vi "803M超标留样MB通讯.vi"(8 "error in (no error)":errorcluster, 9 "VISA resource name":refnum<visa-resource-name> caption="VISA资源名称", 10 "data_in":T1, 11 "功能输入":T2(ring)) -> (0 "error out":errorcluster, 2 "data_out":cluster{"Registers":u16[], "Coils":bool[]})   [LabVIEW 2016, in "超标留样集成.lvlib" / "德润DR803M超标留样.lvlib"]
uses:
  <vilib>/Plasmionique/MB Master/MB_Master_Serial/MB_Master_Serial.lvclass
  D:/Program Files (x86)/National Instruments/LabVIEW 2016/vi.lib/Plasmionique/MB Master/MB_Master/MB_Master.lvclass
  <vilib>/Plasmionique/MB Master/MB Master.lvlib
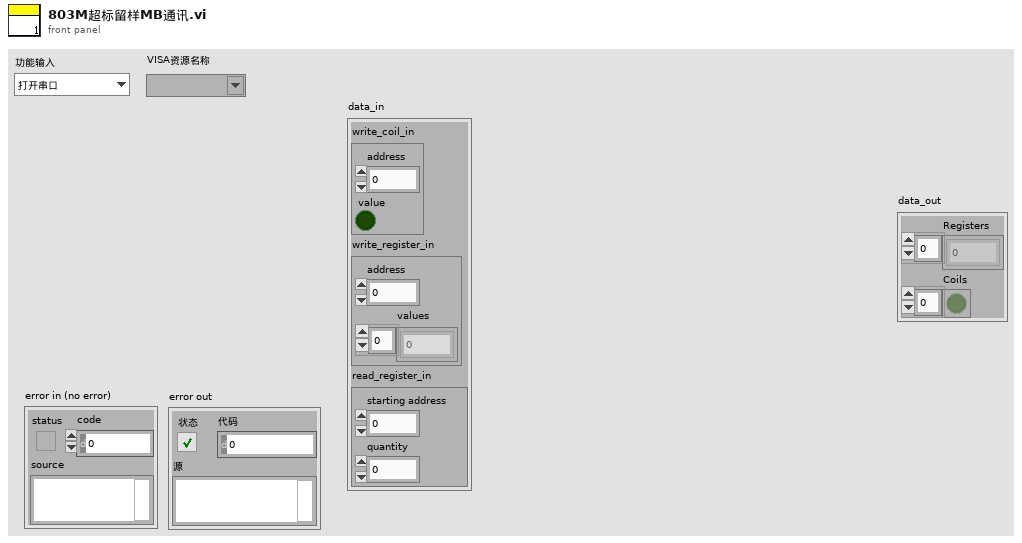
[diagram p1: front panel]
types:
  T1 = cluster{"write_coil_in":cluster{"address":u16, "value":bool}, "write_register_in":cluster{"address":u16, "values":u16[]}, "read_register_in":cluster{"starting address":u16, "quantity":u16}}
  T2 = enum16{"打开串口", "写入", "读取", "关闭串口", "写入寄存器", "读取线圈"}
  T3 = cluster{"baud rate (bps)":u32, "stop bits":u16, "parity":u16, "flow control":u16, "timeout":u32, "retries":i32}
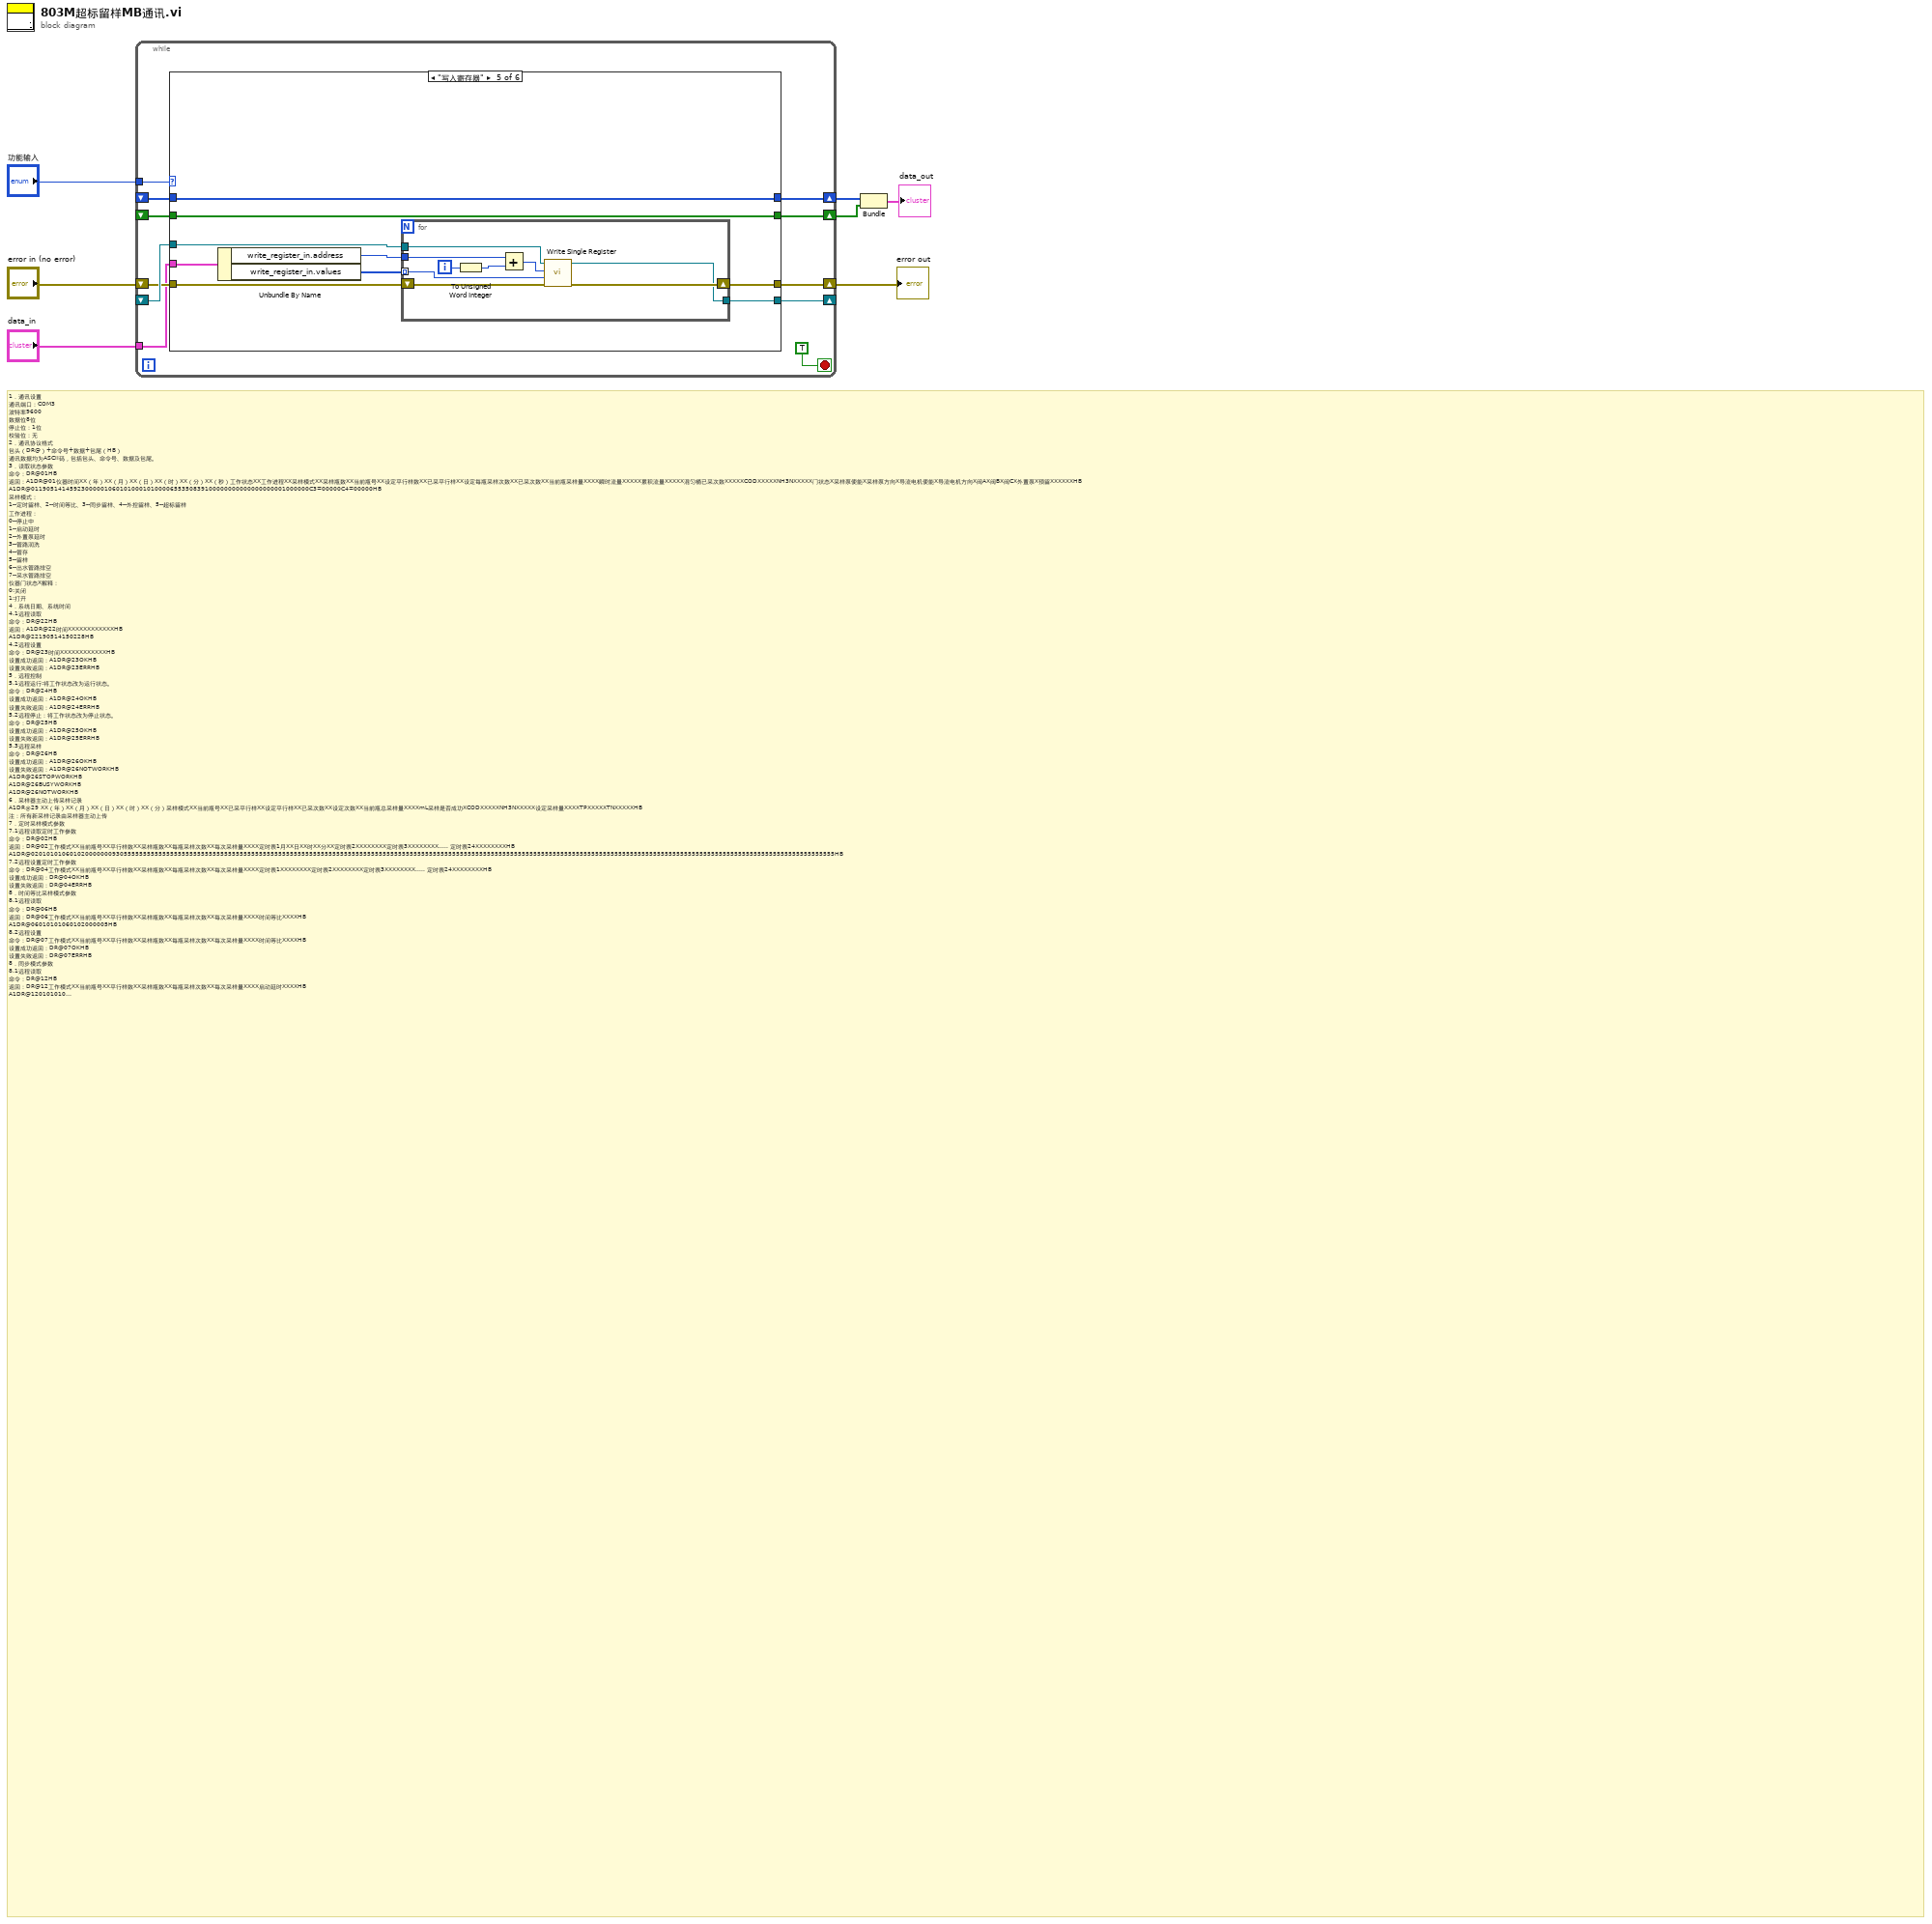
[diagram p0: block diagram]
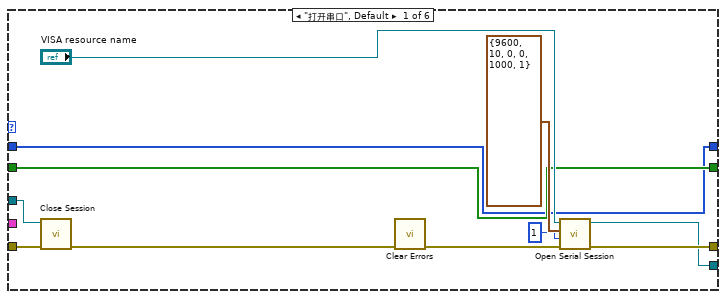
[diagram p2: hidden frame]
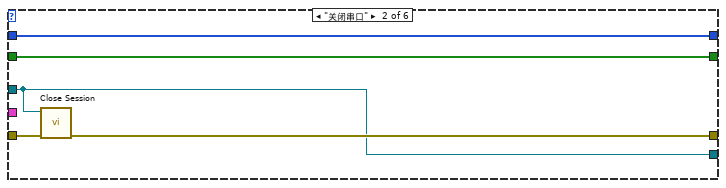
[diagram p3: hidden frame]
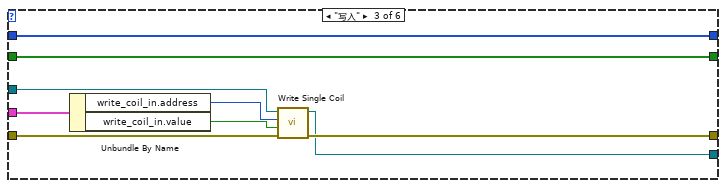
[diagram p4: hidden frame]
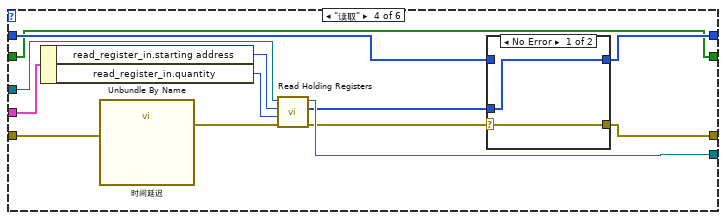
[diagram p5: hidden frame]
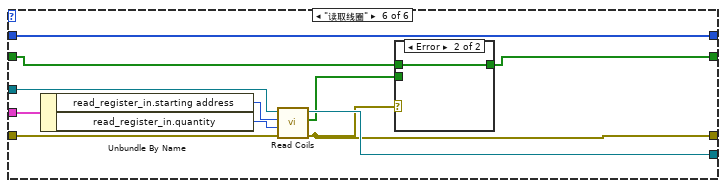
[diagram p7: hidden frame]
diagram:
  # "1．通讯设置\n通讯端口：COM3\n波特率9600 \n数据位8位\n停止位：1位\n校验位：无\n2．通讯协议格式\n包头（DR@）+命令号+数据+包尾（HB）\n通讯数据均为ASCII码，包括包头、命令号、数据及包尾。\n3．读取状态参数\n命令：DR@01HB\n返回：A1DR@01仪器时间XX（年）XX（月）XX（日）XX（时）XX（分）XX（秒）工作状态XX工作进程XX采样模式XX采样瓶数XX当前瓶号XX设定平行样数XX已采平行样XX设定每瓶采样次数XX已采次数XX当前瓶采样量XXXX瞬时流量XXXXX累积流量XXXXX混匀桶已采次数XXXXXCODXXXXXNH3NXXXXX门状态X采样泵使能X采样泵方向X导流电机使能X导流电机方向X阀AX阀BX阀CX外置泵X预留XXXXXXHB\nA1DR@011905141459230000010601010001010000655350839100000000000000000001000000C3=00000C4=00000HB\n采样模式：\n1--定时留样、2--时间等比、3--同步留样、4--外控留样、5--超标留样\n工作进程：\n0--停止中\n1--启动延时\n2--外置泵延时\n3--管路润洗\n4--管存\n5--留样\n6--出水管路排空\n7--采水管路排空\n仪器门状态X解释：\n0:关闭\n1:打开\n4．系统日期、系统时间\n4.1远程读取 \n命令：DR@22HB\n返回：A1DR@22时间XXXXXXXXXXXXHB\nA1DR@22190514150228HB\n4.2远程设置\n命令：DR@23时间XXXXXXXXXXXXHB\n设置成功返回：A1DR@23OKHB\n设置失败返回：A1DR@23ERRHB\n5．远程控制\n5.1远程运行:将工作状态改为运行状态。\n命令：DR@24HB\n设置成功返回：A1DR@24OKHB\n设置失败返回：A1DR@24ERRHB\n5.2远程停止：将工作状态改为停止状态。\n命令：DR@25HB\n设置成功返回：A1DR@25OKHB\n设置失败返回：A1DR@25ERRHB\n5.3远程采样\n命令：DR@26HB\n设置成功返回：A1DR@26OKHB\n设置失败返回：A1DR@26NOTWORKHB\nA1DR@26STOPWORKHB\nA1DR@26BUSYWORKHB\nA1DR@26NOTWORKHB\n6．采样器主动上传采样记录\nA1DR＠29 XX（年）XX（月）XX（日）XX（时）XX（分）采样模式XX当前瓶号XX已采平行样XX设定平行样XX已采次数XX设定次数XX当前瓶总采样量XXXXmL采样是否成功XCODXXXXXNH3NXXXXX设定采样量XXXXTPXXXXXTNXXXXXHB\n注：所有新采样记录由采样器主动上传\n7．定时采样模式参数\n7.1远程读取定时工作参数\n命令：DR@02HB\n返回：DR@02工作模式XX当前瓶号XX平行样数XX采样瓶数XX每瓶采样次数XX每次采样量XXXX定时表1月XX日XX时XX分XX定时表2XXXXXXXX定时表3XXXXXXXX..... 定时表24XXXXXXXXHB\nA1DR@0201010106010200000009305555555555555555555555555555555555555555555555555555555555555555555555555555555555555555555555555555555555555555555555555555555555555555555555555555555555555555555555555555555555555555HB\n7.2远程设置定时工作参数\n命令：DR@04工作模式XX当前瓶号XX平行样数XX采样瓶数XX每瓶采样次数XX每次采样量XXXX定时表1XXXXXXXX定时表2XXXXXXXX定时表3XXXXXXXX..... 定时表24XXXXXXXXHB\n设置成功返回：DR@04OKHB\n设置失败返回：DR@04ERRHB\n8．时间等比采样模式参数\n8.1远程读取\n命令：DR@06HB\n返回：DR@06工作模式XX当前瓶号XX平行样数XX采样瓶数XX每瓶采样次数XX每次采样量XXXX时间等比XXXXHB\nA1DR@06010101060102000005HB\n8.2远程设置\n命令：DR@07工作模式XX当前瓶号XX平行样数XX采样瓶数XX每瓶采样次数XX每次采样量XXXX时间等比XXXXHB\n设置成功返回：DR@07OKHB\n设置失败返回：DR@07ERRHB\n8．同步模式参数\n8.1远程读取\n命令：DR@12HB\n返回：DR@12工作模式XX当前瓶号XX平行样数XX采样瓶数XX每瓶采样次数XX每次采样量XXXX启动延时XXXXHB\nA1DR@12010101060102000010HB\n8.2远程设置\n命令：DR@13工作模式XX当前瓶号XX平行样数XX采样瓶数XX每瓶采样次数XX每次采样量XXXX启动延时XXXXHB\n设置成功返回：DR@13OKHB\n设置失败返回：DR@13ERRHB\n9. 外控留样模式参数\n9.1远程读取\n命令：DR@58HB\n返回：DR@58工作模式XX当前瓶号XX平行样数XX采样瓶数XX每瓶采样次数XX每次采样量XXXXHB\nA1DR@5801010106010200HB\n9.2远程设置\nDR@59工作模式XX当前瓶号XX平行样数XX采样瓶数XX每瓶采样次数XX每次采样量XXXXHB\n设置成功返回：DR@59OKHB\n设置失败返回：DR@59ERRHB\n10．超标模式参数\n10.1远程读取\n命令：DR@16\n返回：DR@16工作模式XX当前瓶号XX平行样数XX采样瓶数XX每瓶采样次数XX每次采样量XXXX采样间隔时间XXXXCOD联机方式XX4mA浓度XXXXX 20mA浓度XXXXX超标浓度XXXXX当前浓度浓度XXXXX NH3N联机方式XX4mA浓度XXXXX 20mA浓度XXXXX超标浓度XXXXX当前浓度浓度XXXXXHB\nA1DR@1605010106010200000503000001000001000000000300000010000010000000HB\n10.2远程设置\n命令：DR@17工作模式XX当前瓶号XX平行样数XX采样瓶数XX每瓶采样次数XX每次采样量XXXX采样间隔XXXXCOD联机方式XX NH3N联机方式XX  COD4mA浓度XXXXX 20mA浓度XXXXX超标浓度XXXXX NH3N 4mA浓度XXXXX 20mA浓度XXXXX超标浓度XXXXX HB\n设置成功返回：DR@17OKHB\n设置失败返回：DR@17ERRHB"
  n1 = while {
    shift-right: [w17] -> _
    shift-left: _ -> [w15]
    shift-right: [w16] -> w5
    shift-left: "error in (no error)" -> [w14]
    tunnel: "功能输入" -> [w13]
    tunnel: "data_in" -> [w12]
    shift-right: [w11] -> w3
    shift-left: _ -> [w10]
    shift-right: [w9] -> w2
    shift-left: _ -> [w8]
    stop <- TRUE stop-if-true
    n2 = case shown="\"写入寄存器\"" w13 {
      tunnel: [w21 w32 w40 w52 w66 w85] -> w17
      tunnel: [w22 w33 w42 w55 w67 w82] -> w16
      tunnel: w15 -> [w28 w32 w41 w54 w69 w88]
      tunnel: w14 -> [w29 w34 w43 w56 w68 w86]
      tunnel: w12 -> [_ _ w37 w47 w65 w84]
      tunnel: [w19 w31 w36 w46 w63 w83] -> w11
      tunnel: w10 -> [w19 w31 w36 w45 w63 w83]
      tunnel: [w20 w30 w35 w44 w64 w80] -> w9
      tunnel: w8 -> [w20 w30 w35 w44 w64 w79]
      frame "打开串口", Default {
        n3 = call-dynamic "Close Session.vi"("error in (no error)"=w29, "MB_Serial session"=w28) -> ("error out"=w27:errorcluster)  [unwired: 9 in]
        n4 = call <vilib>:"Clear Errors.vi"("error in (no error)"=w27) -> ("error out"=w23:errorcluster)  [unwired: 5 in, 1 out]
        n5 = call <vilib>:"Open Serial Session.vi"("Error in"=w23, "Slave ID"=u8 1, "Serial Config"=T3 {"baud rate (bps)"=9600, "stop bits"=10, "parity"=0, "flow control"=0, "timeout"=1000, "retries"=1}, "VISA Resource"="VISA resource name") -> ("Error out"=w22:errorcluster, "MB_Serial session"=w21:refnum<class "MB_Master_Serial.lvclass">)  [unwired: 6 in]
      }
      frame "关闭串口" {
        n6 = call-dynamic "Close Session.vi"("error in (no error)"=w34, "MB_Serial session"=w32) -> ("error out"=w33:errorcluster)  [unwired: 9 in]
      }
      frame "写入" {
        n7 = Unbundle By Name(w37) -> ("write_coil_in.address"=w39:u16, "write_coil_in.value"=w38:bool)
        n8 = call <vilib>:"Write Single Coil.vi"("error in (no error)"=w43, "value"=w38, "address"=w39, "MB session in"=w41) -> ("error out"=w42:errorcluster, "MB session out"=w40:refnum<class "MB_Master_Serial.lvclass">)  [unwired: 6 in]
      }
      frame "读取" {
        n9 = Unbundle By Name(w47) -> ("read_register_in.starting address"=w49:u16, "read_register_in.quantity"=w48:u16)
        n10 = call "时间延迟"("error in (no error)"=w56) -> ("error out"=w53:errorcluster)  [unwired: 10 in]
        n11 = call <vilib>:"Read Holding Registers.vi"("error in (no error)"=w53, "quantity"=w48, "starting address"=w49, "MB session in"=w54) -> ("error out"=w51:errorcluster, "Registers"=w50:u16[], "MB session out"=w52:refnum<class "MB_Master_Serial.lvclass">)  [unwired: 5 in]
        n12 = case shown="No Error" w51 {
          selector: w51 -> [w58 w60]
          tunnel: [w58 w60] -> w55
          tunnel: w50 -> [w57 _]
          tunnel: [w57 w59] -> w46
          tunnel: w45 -> [_ w59]
          frame No Error {
          }
          frame Error {
          }
        }
      }
      frame "写入寄存器" {
        n13 = Unbundle By Name(w65) -> ("write_register_in.address"=w62:u16, "write_register_in.values"=w61:u16[])
        n14 = for {
          tunnel: w69 -> [w78]
          tunnel: [w75] -> w66
          shift-right: [w76] -> w67
          shift-left: w68 -> [w77]
          tunnel: w62 -> [w74]
          tunnel: w61 -> [w70] mode=indexing
          i -> [w73]
          n15 = To Unsigned Word Integer(number=w73) -> (unsigned 16bit integer=w71:u16)
          n16 = Add(x=w74, y=w71) -> (x+y=w72:u16)
          n17 = call <vilib>:"Write Single Register.vi"("error in (no error)"=w77, "value"=w70, "address"=w72, "MB session in"=w78) -> ("error out"=w76:errorcluster, "MB session out"=w75:refnum<class "MB_Master_Serial.lvclass">)  [unwired: 6 in]
        }
      }
      frame "读取线圈" {
        n18 = Unbundle By Name(w84) -> ("read_register_in.starting address"=w89:u16, "read_register_in.quantity"=w87:u16)
        n19 = call <vilib>:"Read Coils.vi"("error in (no error)"=w86, "quantity"=w87, "starting address"=w89, "MB session in"=w88) -> ("error out"=w82:errorcluster, "Coils"=w81:bool[], "MB session out"=w85:refnum<class "MB_Master_Serial.lvclass">)  [unwired: 5 in]
        n20 = case shown="Error" w82 {
          tunnel: w81 -> [w90 _]
          tunnel: [w90 w91] -> w80
          tunnel: w79 -> [_ w91]
          frame No Error {
          }
          frame Error {
          }
        }
      }
    }
  }
  "error out" <- w5
  n21 = Bundle("Registers"=w3, "Coils"=w2) -> (→"data_out":cluster{"Registers":u16[], "Coils":bool[]})  [unwired: 1 in]
